vi "Set_CHROMA.vi"(3 "instrument handle out":refnum<k15>) -> (11 "instrument handle":refnum<k15>)   [LabVIEW 2012]
uses:
  FT_HMI.llb/GLOBAL_GEN.vi
  FT_HMI.llb/GLOBAL_PUMPS_PARAMS.vi
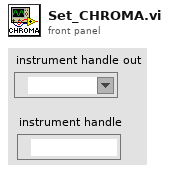
[diagram p1: front panel]
types:
  T1 = cluster{"VAC":cluster{"ENABLE":bool, "PUMPING_TIME [ms]":dbl, "MEASUREMENT_TIME [ms]":dbl, "PRESSURE_LIMIT [bar]":sgl}, "Q1":cluster{"ENABLE":bool, "PUMPING_TIME  [ms]":dbl, "MEASUREMENT_TIME  [ms]":sgl, "FLOW_TARGET  [ml/min]":sgl, "FLOW_LIMIT_UP  [ml/min]":sgl, "FLOW_LIMIT_DOWN [ml/min]":sgl, "PRESSURE_TARGET [bar]":sgl, "PRESSURE_LIMIT_UP [bar]":sgl, "PRESSURE_LIMIT_DOWN [bar]":sgl, "MAX_FLOW":bool}, "Q2":cluster{"ENABLE":bool, "PUMPING_TIME [ms]":dbl, "MEASUREMENT_TIME [ms]":dbl, "FLOW_TARGET [ml/min]":sgl, "FLOW_LIMIT_UP [ml/min]":sgl, "FLOW_LIMIT_DOWN [ml/min]":sgl, "PRESSURE_TARGET [bar]":sgl, "PRESSURE_LIMIT_UP [bar]":sgl, "PRESSURE_LIMIT_DOWN [bar]":sgl, "MAX_FLOW":bool}, "PMAX":cluster{"ENABLE":bool, "PUMPING_TIME [ms]":dbl, "MEASUREMENT_TIME [ms]":dbl, "PRESSURE_LIMIT [bar]":sgl, "PRESSURE_LOOSE_TIME [ms]":sgl}, "PRINT":cluster{"ENABLE":bool}, "SUPPLY":cluster{"VOLTAGE [V]":dbl, "FREQUENCY [Hz]":dbl}}
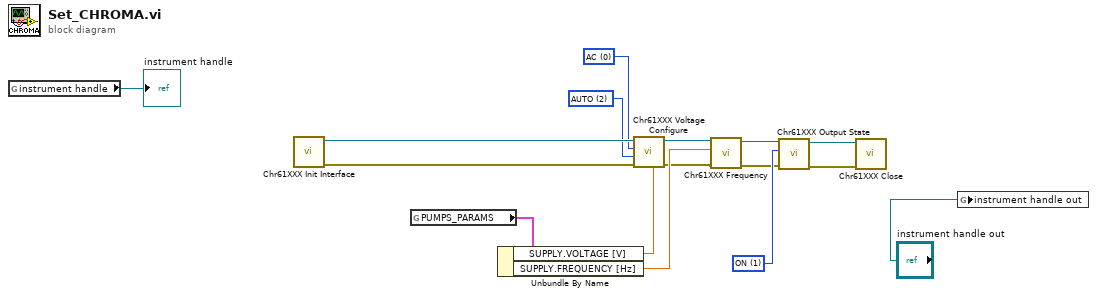
[diagram p0: block diagram]
diagram:
  w10 = 2 items=["LOW", "HIGH", "AUTO"] ("voltage range")
  w9 = 0 items=["AC", "DC"] ("voltage type")
  w6 = u16 1 items=["OFF", "ON"] ("state")
  n1 = global read "GLOBAL_GEN.vi" "instrument handle"() -> (→"instrument handle":refnum<k15>)
  n2 = call <instrlib>:"Chr61XXX Init Interface.vi"() -> ("error out"=w11:errorcluster, "instrument handle out"=w12:refnum<k15>)  [unwired: 9 in, 1 out]
  n3 = global read "GLOBAL_PUMPS_PARAMS.vi" "PUMPS_PARAMS"() -> (w3:T1)
  n4 = Unbundle By Name(w3) -> ("SUPPLY.VOLTAGE [V]"=w5:dbl, "SUPPLY.FREQUENCY [Hz]"=w4:dbl)
  n5 = call <instrlib>:"Chr61XXX Voltage Configure.vi"("voltage"=w5, "error in (no error)"=w11, "voltage range"=w10, "voltage type"=w9, "instrument handle"=w12) -> ("error out"=w2:errorcluster, "instrument handle out"=w8:refnum<k15>)  [unwired: 5 in]
  n6 = call <instrlib>:"Chr61XXX Frequency.vi"("error in (no error)"=w2, "frequency"=w4, "instrument handle"=w8) -> ("error out"=w1:errorcluster, "instrument handle out"=w7:refnum<k15>)  [unwired: 7 in]
  n7 = call <instrlib>:"Chr61XXX Output State.vi"("error in (no error)"=w1, "state"=w6, "instrument handle"=w7) -> ("error out"=w13:errorcluster, "instrument handle out"=w16:refnum<k15>)  [unwired: 7 in]
  n8 = call <instrlib>:"Chr61XXX Close.vi"("error in (no error)"=w13, "instrument handle"=w16) -> ()  [unwired: 9 in, 1 out]
  n9 = global write "GLOBAL_GEN.vi" "instrument handle out"("instrument handle out") -> ()
